vi "elapsed_time.vi"(7 "Command":T1, 8 "error in (no error)":errorcluster, 11 "Desired Time (s)":u32) -> (0 "error out":errorcluster, 2 "Is Done?":bool, 3 "Elapsed Time":dbl)   [LabVIEW 2017]
uses:
  controls/ElapsedTimeCmd.ctl
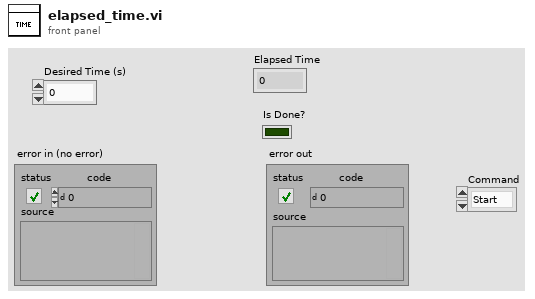
[diagram p1: front panel]
types:
  T1 = typedef "ElapsedTimeCmd.ctl" = enum16{"Start", "Stop", "Check Time"}
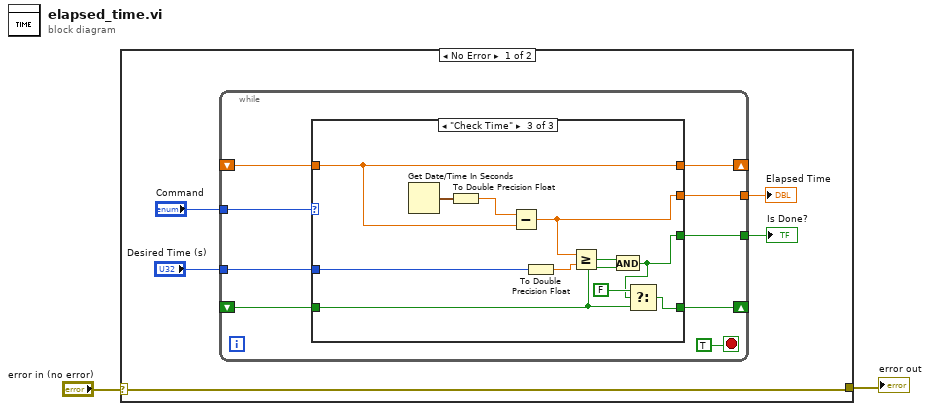
[diagram p0: block diagram]
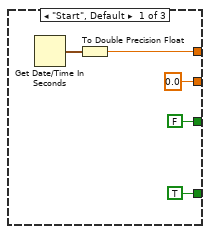
[diagram p2: hidden frame]
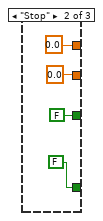
[diagram p3: hidden frame]
diagram:
  n1 = case shown="No Error" "error in (no error)" {
    selector: "error in (no error)" -> [w7 w37]
    tunnel: [w7 w37] -> w1
    frame No Error {
      n2 = while {
        tunnel: "Desired Time (s)" -> [w16]
        tunnel: [w15] -> w5
        tunnel: [w14] -> w4
        tunnel: "Command" -> [w13]
        shift-right: [w12] -> _
        shift-left: _ -> [w11]
        shift-right: [w10] -> _
        shift-left: _ -> [w9]
        stop <- TRUE stop-if-true
        n3 = case shown="\"Check Time\"" w13 {
          tunnel: w16 -> [_ _ w33]
          tunnel: [0.0 0.0 w32] -> w15
          tunnel: [FALSE FALSE ("Is Done?") w26] -> w14
          tunnel: [w20 0.0 w34] -> w12
          tunnel: w11 -> [_ _ w34]
          tunnel: [TRUE FALSE ("Is Done?") w28] -> w10
          tunnel: w9 -> [_ _ w27]
          frame "Start", Default {
            n4 = Get Date/Time In Seconds() -> (seconds since 1Jan1904=w21:timestamp)
            n5 = To Double Precision Float(number=w21) -> (double precision float=w20:dbl)
          }
          frame "Stop" {
          }
          frame "Check Time" {
            n6 = Get Date/Time In Seconds() -> (seconds since 1Jan1904=w36:timestamp)
            n7 = To Double Precision Float(number=w36) -> (double precision float=w35:dbl)
            n8 = Subtract(x=w35, y=w34) -> (x-y=w32:dbl)
            n9 = To Double Precision Float(number=w33) -> (double precision float=w31:dbl)
            n10 = Greater Or Equal?(x=w32, y=w31) -> (x >= y?=w30:bool)
            n11 = And(x=w30, y=w27) -> (x .and. y?=w26:bool)
            n12 = Select(t=FALSE, s=w26, f=w27) -> (s? t:f=w28:bool)
          }
        }
      }
      "Elapsed Time" <- w5
      "Is Done?" <- w4
    }
    frame Error {
    }
  }
  "error out" <- w1
